vi "AMZ_S3_APIHLP_Parse BucketLoggingStatus.vi"(8 "error in (no error)":errorcluster, 10 "Response body":string) -> (0 "error out":errorcluster, 3 "BucketLoggingStatus":T1)   [LabVIEW 2015, in "LV Interface for Amazon S3.lvlib"]
uses:
  LV Interface for Amazon S3.lvlib
  Typedefs/AMZ_S3_API_BucketLoggingStatus.ctl
  Typedefs/AMZ_S3_Grant.ctl
  Typedefs/AMZ_S3_Grantee.ctl
  Typedefs/AMZ_S3_LoggingPermission.ctl
  XML Parser/XML Parser.lvlib
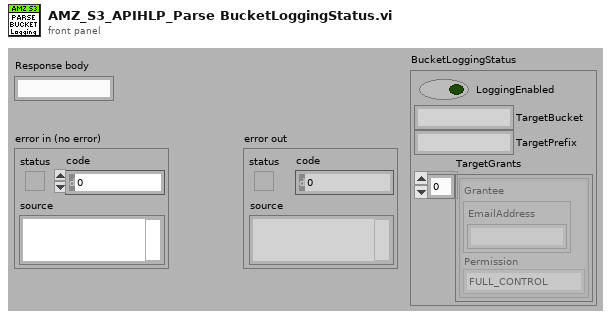
[diagram p1: front panel]
types:
  T1 = typedef "LV Interface for Amazon S3.lvlib/AMZ_S3_API_BucketLoggingStatus.ctl" = cluster{"LoggingEnabled":bool, "TargetBucket":string, "TargetPrefix":string, "TargetGrants":T2[]}
  T2 = typedef "LV Interface for Amazon S3.lvlib/AMZ_S3_Grant.ctl" = cluster{"Grantee":T3, "Permission":T4}
  T3 = typedef "LV Interface for Amazon S3.lvlib/AMZ_S3_Grantee.ctl" = cluster{"EmailAddress":string}
  T4 = typedef "LV Interface for Amazon S3.lvlib/AMZ_S3_LoggingPermission.ctl" = enum16{"FULL_CONTROL", "READ", "WRITE"}
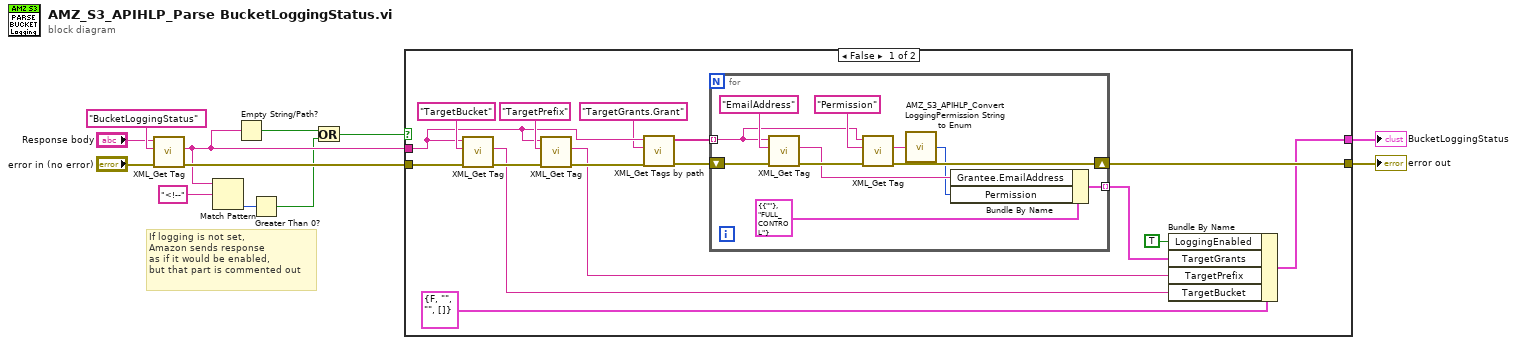
[diagram p0: block diagram]
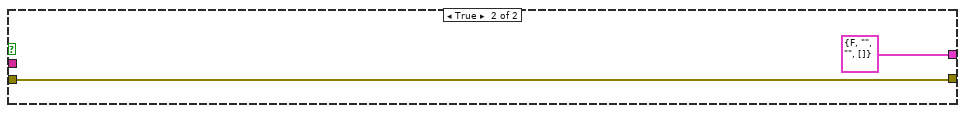
[diagram p2: hidden frame]
diagram:
  # "If logging is not set,\nAmazon sends response\nas if it would be enabled,\nbut that part is commented out"
  n1 = call "XML_Get Tag.vi"("error in (no error)"="error in (no error)", "Tag name"="BucketLoggingStatus", "XML String in"="Response body") -> ("error out"=w9:errorcluster, "Tag value"=w6:string)  [unwired: 4 in, 3 out]
  n2 = Match Pattern(string=w6, regular expression="<!--") -> (offset past match=w4:i32)  [unwired: 1 in, 3 out]
  n3 = Empty String/Path?(string/path=w6) -> (empty?=w3:bool)
  n4 = Greater Than 0?(x=w4) -> (x > 0?=w2:bool)
  n5 = Or(x=w3, y=w2) -> (x .or. y?=w1:bool)
  n6 = case shown="False" w1 {
    tunnel: w6 -> [w23 _]
    tunnel: w9 -> [w28 w41]
    tunnel: [w14 w41] -> w7
    tunnel: [w13 T1 {"LoggingEnabled"=FALSE, "TargetBucket"="", "TargetPrefix"="", "TargetGrants"=[]} ("BucketLoggingStatus")] -> w8
    frame False {
      n7 = call "XML_Get Tag.vi"("error in (no error)"=w28, "Tag name"="TargetBucket", "XML String in"=w23) -> ("error out"=w26:errorcluster, "Tag value"=w17:string)  [unwired: 4 in, 3 out]
      n8 = call "XML_Get Tag.vi"("error in (no error)"=w26, "Tag name"="TargetPrefix", "XML String in"=w23) -> ("error out"=w24:errorcluster, "Tag value"=w16:string)  [unwired: 4 in, 3 out]
      n9 = call "XML_Get Tags by path.vi"("error in (no error)"=w24, "Tag path"="TargetGrants.Grant" ("Tag name"), "XML String in"=w23) -> ("error out"=w21:errorcluster, "Matching tag values"=w20:string[])  [unwired: 7 in]
      n10 = for {
        shift-right: [w34] -> w14
        shift-left: w21 -> [w39]
        tunnel: w20 -> [w36] mode=indexing
        tunnel: [w29] -> w18 mode=indexing
        n11 = call "XML_Get Tag.vi"("error in (no error)"=w39, "Tag name"="EmailAddress", "XML String in"=w36) -> ("error out"=w35:errorcluster, "Tag value"=w32:string)  [unwired: 4 in, 3 out]
        n12 = call "XML_Get Tag.vi"("error in (no error)"=w35, "Tag name"="Permission", "XML String in"=w36) -> ("error out"=w34:errorcluster, "Tag value"=w31:string)  [unwired: 4 in, 3 out]
        n13 = call "AMZ_S3_APIHLP_Convert LoggingPermission String to Enum.vi"("LoggingPermission String"=w31) -> ("Permission"=w30:T4)  [unwired: 4 in]
        n14 = Bundle By Name(cluster=T2 {"Grantee"={"EmailAddress"=""}, "Permission"=enum."FULL_CONTROL"} ("Grant"), "Grantee.EmailAddress"=w32, "Permission"=w30) -> (w29:T2)
      }
      n15 = Bundle By Name(cluster=T1 {"LoggingEnabled"=FALSE, "TargetBucket"="", "TargetPrefix"="", "TargetGrants"=[]} ("BucketLoggingStatus"), "LoggingEnabled"=TRUE, "TargetGrants"=w18, "TargetPrefix"=w16, "TargetBucket"=w17) -> (w13:T1)
    }
    frame True {
    }
  }
  "error out" <- w7
  "BucketLoggingStatus" <- w8
